vi "Get Input Channel Registers.vi"(8 "error in (no error)":errorcluster, 11 "Input Channels":T3[](array[typedef]) format="%.0x") -> (0 "error out":errorcluster, 3 "Input Register Info":T2(array[cluster]))   [LabVIEW 2010, in "Sensor Simulation Custom Device.lvlib"]
uses:
  Sensor Simulation Custom Device.lvlib
  <vilib>/NI Veristand/Custom Device API/Custom Device Item Ref.ctl
  TypeDefs/InputChannelTypes.ctl
  <vilib>/NI Veristand/Custom Device API/Custom Device API.lvlib
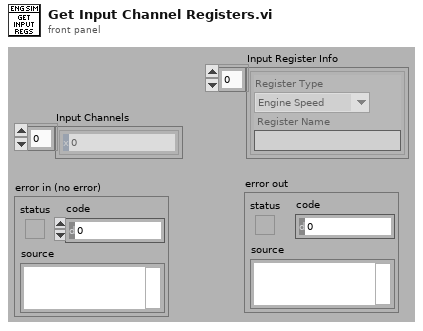
[diagram p1: front panel]
types:
  T1 = typedef "Sensor Simulation Custom Device.lvlib/InputChannelTypes.ctl" = enum16{"Engine Speed", "Offset"}
  T2 = cluster{"Register Type":T1, "Register Name":string}[]
  T3 = typedef "Custom Device API.lvlib/Custom Device Item Ref.ctl" = u64
  T4 = typedef "Custom Device API.lvlib/Custom Device Item Info.ctl" = cluster{"Name":string, "Is Channel":bool, "GUID":string}
  T5 = cluster{"Output Channel Types":T1, "string":string}
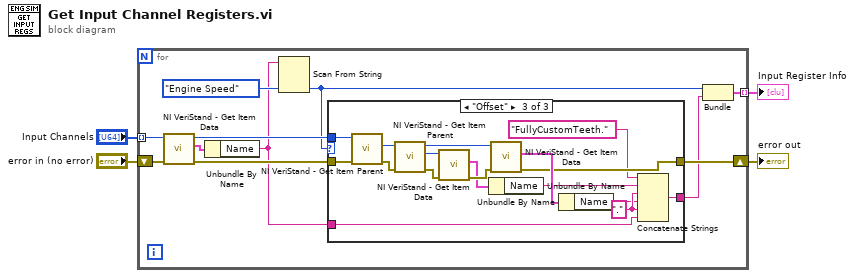
[diagram p0: block diagram]
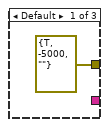
[diagram p2: hidden frame]
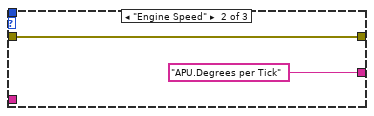
[diagram p3: hidden frame]
diagram:
  n1 = for {
    tunnel: "Input Channels" -> [w15] mode=indexing
    shift-right: [w10] -> w4
    shift-left: "error in (no error)" -> [w11]
    tunnel: [w6] -> w2 mode=indexing
    n2 = call <vilib>:"NI VeriStand - Get Item Data.vi"("error in (no error)"=w11, "Item Ref in"=w15) -> ("error out"=w12:errorcluster, "Item Info"=w14:T4, "Item Ref out"=w13:T3)  [unwired: 6 in, 1 out]
    n3 = Unbundle By Name(w14) -> ("Name"=w7:string)
    n4 = Scan From String(input string=w7, default 1=InputChannelTypes."Engine Speed" ("Output Channel Types")) -> (output 1=w8:T1)  [unwired: 3 in, 3 out]
    n5 = case shown="\"Offset\"" w8 {
      tunnel: w13 -> [_ _ w35]
      tunnel: w12 -> [_ w18 w34]
      tunnel: [errorcluster {"status"=TRUE, "code"=-5000, "source"=""} ("error out") w18 w25] -> w10
      tunnel: [_ "APU.Degrees per Tick" ("string") w22] -> w5
      tunnel: w7 -> [_ _ w21]
      frame Default {
      }
      frame "Engine Speed" {
      }
      frame "Offset" {
        w23 = "." ("string")
        n6 = call <vilib>:"NI VeriStand - Get Item Parent.vi"("error in (no error)"=w34, "Item Ref in"=w35) -> ("error out"=w32:errorcluster, "Parent Ref"=w33:T3)  [unwired: 6 in, 2 out]
        n7 = call <vilib>:"NI VeriStand - Get Item Parent.vi"("error in (no error)"=w32, "Item Ref in"=w33) -> ("error out"=w30:errorcluster, "Parent Ref"=w31:T3, "Item Ref out"=w29:T3)  [unwired: 6 in, 1 out]
        n8 = call <vilib>:"NI VeriStand - Get Item Data.vi"("error in (no error)"=w30, "Item Ref in"=w31) -> ("error out"=w28:errorcluster, "Item Info"=w27:T4)  [unwired: 6 in, 2 out]
        n9 = Unbundle By Name(w27) -> ("Name"=w19:string)
        n10 = call <vilib>:"NI VeriStand - Get Item Data.vi"("error in (no error)"=w28, "Item Ref in"=w29) -> ("error out"=w25:errorcluster, "Item Info"=w26:T4)  [unwired: 6 in, 2 out]
        n11 = Unbundle By Name(w26) -> ("Name"=w20:string)
        n12 = Concatenate Strings("FullyCustomTeeth." ("string"), w19, w23, w20, w23, w21) -> (w22:string)
      }
    }
    n13 = Bundle("Output Channel Types"=w8, "string"=w5) -> (w6:T5)  [unwired: 1 in]
  }
  "error out" <- w4
  "Input Register Info" <- w2
